vi "User Permissions Cluster to Number.vi"(1 "User Permisions":T1) -> (0 "User Permissions":i32)   [LabVIEW 2011]
uses:
  User Permissions.ctl
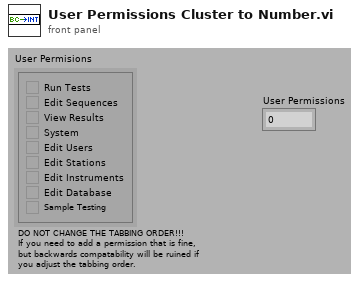
[diagram p1: front panel]
types:
  T1 = typedef "User Permissions.ctl" = cluster{"Run Tests":bool, "Edit Sequences":bool, "View Results":bool, "System":bool, "Edit Users":bool, "Edit Stations":bool, "Edit Instruments":bool, "Edit Database":bool, "Sample Testing":bool}
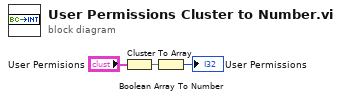
[diagram p0: block diagram]
diagram:
  n1 = Cluster To Array(cluster="User Permisions") -> (array=w2:bool[])
  n2 = Boolean Array To Number(Boolean array=w2) -> (number=→"User Permissions":u32)
